vi "init_drive_frame.vi"(8 "error in (no error)":errorcluster) -> (0 "error out":errorcluster, 3 "differential steering frame out":refnum<class "NI_Robotics_Differential Steering Frame.lvclass">)   [LabVIEW 2011]
uses:
  <vilib>/robotics/Steering/Differential Steering Frame/NI_Robotics_Differential Steering Frame.lvclass
  <vilib>/robotics/Steering/Wheel/Wheel Parameters.ctl
  <vilib>/robotics/Steering/Wheel/Rotation Direction.ctl
  <vilib>/robotics/Steering/Fixed Wheel/Create Fixed Wheel.vi
  <vilib>/robotics/Steering/Differential Steering Frame/Create Differential Steering Frame.vi
  <vilib>/robotics/Steering/Wheel/NI_Robotics_Wheel.lvclass
  <vilib>/robotics/Steering/Fixed Wheel/NI_Robotics_Fixed Wheel.lvclass
  <vilib>/robotics/Steering/Steering Frame/NI_Robotics_Steering Frame.lvclass
panel:
  # "This VI creates a simple differential-steering frame\nwith the steering API.  This frame will be used in\nthe Navigation Loop."
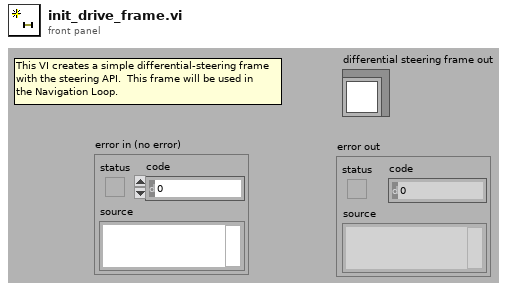
[diagram p1: front panel]
types:
  T1 = typedef "NI_Robotics_Wheel.lvclass/Wheel Parameters.ctl" = cluster{"wheel radius":dbl, "gear ratio":dbl, "forward rotation direction":T2}
  T2 = typedef "NI_Robotics_Wheel.lvclass/Rotation Direction.ctl" = enum16{"Clockwise", "Counterclockwise"}
  T3 = cluster{"fixed wheel out":refnum<class "NI_Robotics_Fixed Wheel.lvclass">, "fixed wheel out":refnum<class "NI_Robotics_Fixed Wheel.lvclass">}
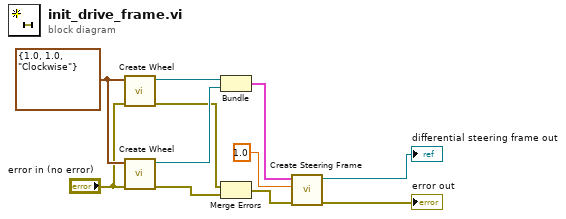
[diagram p0: block diagram]
diagram:
  w11 = T1 {"wheel radius"=1.0, "gear ratio"=1.0, "forward rotation direction"=enum."Clockwise"} ("wheel parameters")
  n1 = call-poly <vilib>:"Create Wheel.vi"("error in (no error)"="error in (no error)", "wheel parameters"=w11) -> ("error out"=w4:errorcluster, "fixed wheel out"=w10:refnum<class "NI_Robotics_Fixed Wheel.lvclass">)  [unwired: 8 in]
  n2 = call-poly <vilib>:"Create Wheel.vi"("error in (no error)"="error in (no error)", "wheel parameters"=w11) -> ("error out"=w3:errorcluster, "fixed wheel out"=w9:refnum<class "NI_Robotics_Fixed Wheel.lvclass">)  [unwired: 8 in]
  n3 = Bundle("fixed wheel out"=w10, "fixed wheel out"=w9) -> (w8:T3)  [unwired: 1 in]
  n4 = Merge Errors(w4, w3) -> (w2:errorcluster)
  n5 = call-poly <vilib>:"Create Steering Frame.vi"("error in (no error)"=w2, "wheel separation"=1.0, "wheels"=w8) -> ("error out"=→"error out":errorcluster, "differential steering frame out"=→"differential steering frame out":refnum<class "NI_Robotics_Differential Steering Frame.lvclass">)  [unwired: 7 in]
